vi "Timed Message_New Interval.vi"(0 "Timed Message In":refnum<class "Timed Message.lvclass">, 7 "New Interval":i32, 11 "error in (no error)":errorcluster) -> (4 "Timed Message Out":refnum<class "Timed Message.lvclass">, 15 "error out":errorcluster)   [LabVIEW 2012, in "Timed Message.lvclass"]
uses:
  Timed Message.lvclass
  src/Connector/FTW-ActorConnector.lvclass
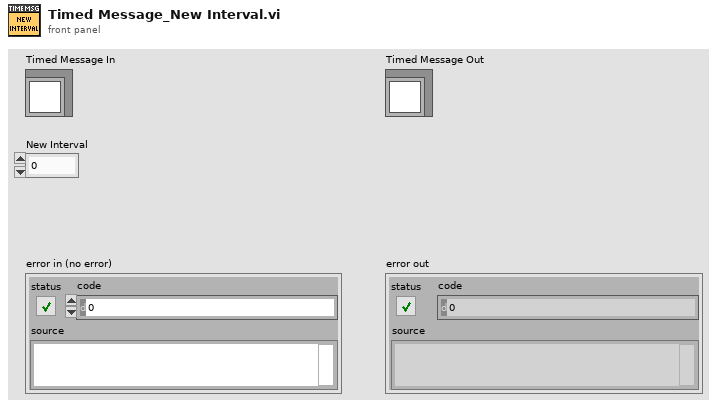
[diagram p1: front panel]
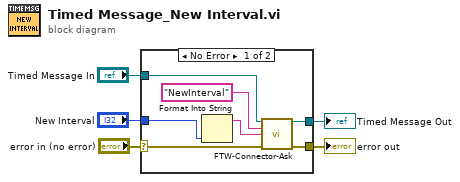
[diagram p0: block diagram]
diagram:
  n1 = case shown="No Error" "error in (no error)" {
    selector: "error in (no error)" -> [w10 w13]
    tunnel: "Timed Message In" -> [w12 w14]
    tunnel: [w11 w14] -> w3
    tunnel: [w9 w13] -> w2
    tunnel: "New Interval" -> [w7 _]
    frame No Error {
      n2 = Format Into String(w7) -> (resulting string=w6:string)  [unwired: 3 in, 1 out]
      n3 = call "FTW-Connector-Ask.vi"("FTW Actor Connector"=w12, "Request Header"="NewInterval", "Request Body"=w6, "error in"=w10) -> ("FTW Actor Connector out"=w11:refnum<class "Timed Message.lvclass">, "error out"=w9:errorcluster)  [unwired: 7 in, 3 out]
    }
    frame Error {
    }
  }
  "Timed Message Out" <- w3
  "error out" <- w2
